vi "draft.vi"() -> ()   [LabVIEW 2017]
panel:
  out "*(type *) &x":string
  out "string":string
  out "size(s)":i32
  out "Array 5":u8[](array[numeric])
  out "Array 4":u8[][](array[numeric])
  out "x = y?":bool
  out "Numeric":i32
  out "array w/ subset deleted":u8[](array[numeric]) format="%.0x"
  out "Array":i32[](array[numeric])
  out "(hi.lo)":u16
  out "Array 3":u8[](array[numeric]) format="%.0x"
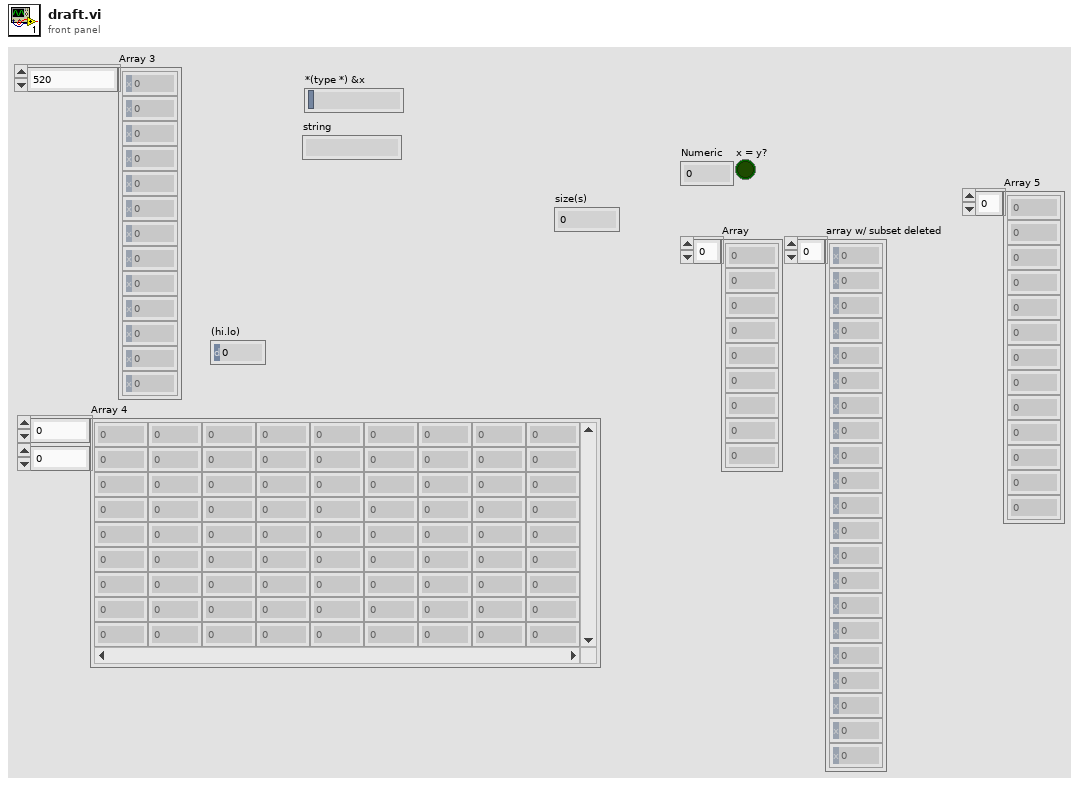
[diagram p1: front panel]
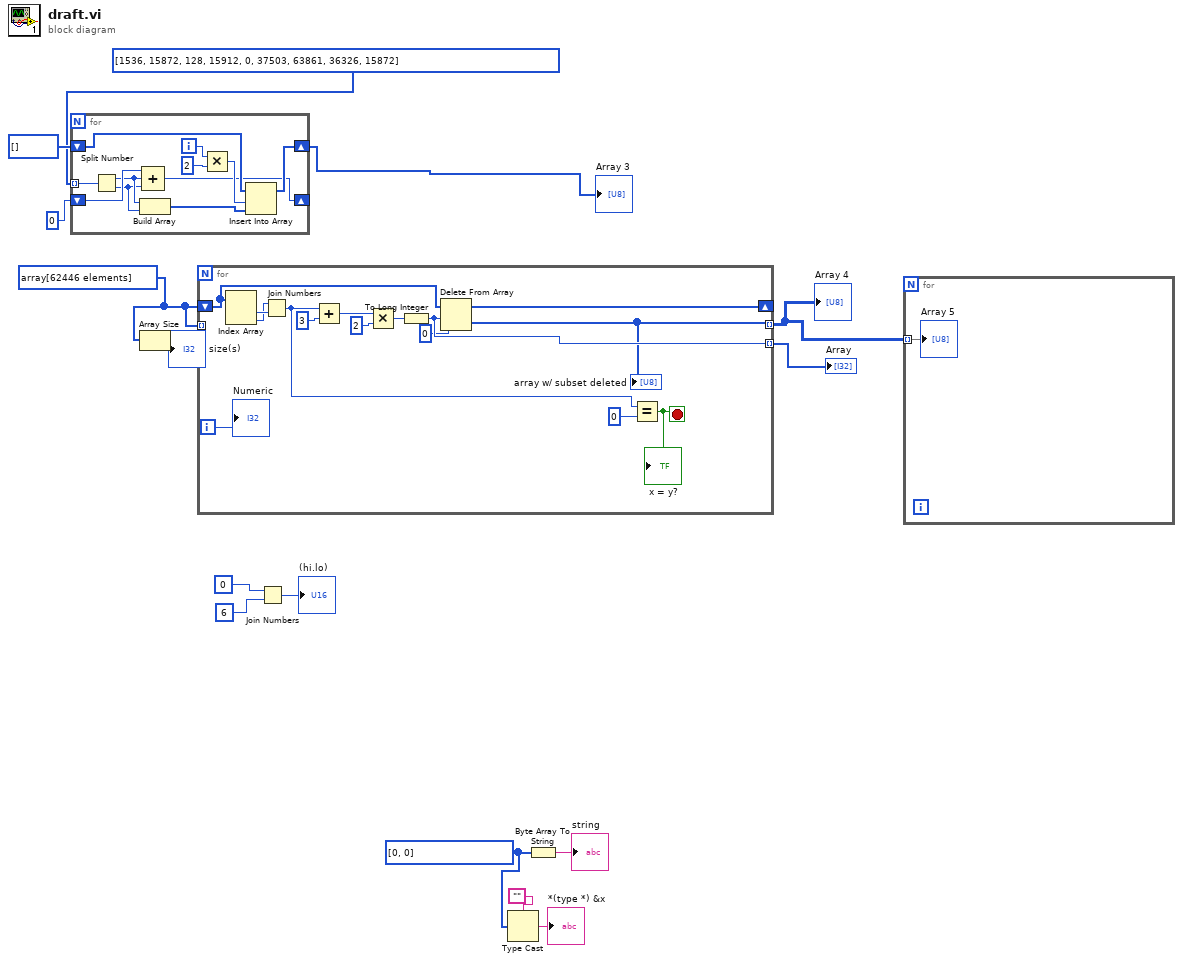
[diagram p0: block diagram]
diagram:
  w3 = u8[] [0, 0] ("unsigned byte array")
  w6 = u8[] array[62446 elements] ("Array 4")
  n1 = for {
    tunnel: u16[] [1536, 15872, 128, 15912, 0, 37503, 63861, 36326, 15872] ("Array 4") -> [w26] mode=indexing
    shift-right: [w21] -> w13
    shift-left: u8[] [] -> [w20]
    shift-right: [w18] -> _
    shift-left: u16 0 -> [w19]
    i -> [w25]
    n2 = Split Number(x=w26) -> (hi(x)=w17:u8, lo(x)=w16:u8)
    n3 = Build Array(w17, w16) -> (w23:u8[])
    n4 = Compound Arithmetic op=ADD(w19, w17, w16) -> (w18:u16)
    n5 = Multiply(x=w25, y=2) -> (x*y=w22:i32)
    n6 = Insert Into Array(array=w20, index=w22, new element=w23) -> (w21:u8[])
  }
  "Array 3" <- w13
  n7 = Array Size(array=w6) -> (size(s)=→"size(s)":i32)
  n8 = for {
    shift-right: [w28] -> _
    shift-left: w6 -> [w41]
    tunnel: [w32] -> w8 mode=indexing
    tunnel: w6 -> [_] mode=indexing
    tunnel: [w27] -> w7 mode=indexing
    i -> [w30]
    stop <- w34 stop-if-true
    n9 = Index Array(array=w41) -> (element #1=w40:u8, element #2=w39:u8)  [unwired: 2 in]
    n10 = Join Numbers(hi=w39, lo=w40) -> ((hi.lo)=w29:u16)
    n11 = Add(x=w29, y=u16 3) -> (x+y=w37:u16)
    n12 = Multiply(x=w37, y=u16 2) -> (x*y=w35:u16)
    n13 = To Long Integer(number=w35) -> (32bit integer=w32:i32)
    n14 = Delete From Array(array=w41, length=w32, index=0) -> (deleted portion=w27:u8[], array with subset deleted=w28:u8[])
    "array w/ subset deleted" <- w27
    n15 = Equal?(x=w29, y=0) -> (x = y?=w34:bool)
    "x = y?" <- w34
    "Numeric" <- w30
  }
  "Array" <- w8
  "Array 4" <- w7
  n16 = Join Numbers(hi=u8 0, lo=u8 6) -> ((hi.lo)=→"(hi.lo)":u16)
  n17 = Type Cast(type="", x=w3) -> (*(type *) &x=→"*(type *) &x":string)
  n18 = Byte Array To String(unsigned byte array=w3) -> (string=→"string":string)
  n19 = for {
    tunnel: w7 -> [w42] mode=indexing
    "Array 5" <- w42
  }
